vi "Action.vi"(8 "error in (no error)":errorcluster, 10 "OOQMH in":refnum<class "OOQMH.lvclass">, 11 "Get Notifiers in":refnum<class "Get Notifiers.lvclass">) -> (0 "error out":errorcluster, 2 "OOQMH out":refnum<class "OOQMH.lvclass">, 3 "Get Notifiers out":refnum<class "Get Notifiers.lvclass">)   [LabVIEW 2024, in "PID Loop.lvlib" / "Get Notifiers.lvclass"]
uses:
  Get Notifiers.lvclass
  Get Notifiers.lvclass/Get Notifiers.ctl
  PID Loop/PID Loop.lvclass
  C:/Users/uspoaotto/OneDrive - Oregon Tool/Desktop/working copies/helperLoop/src/OOQMH/OOQMH/OOQMH.lvclass
  C:/Users/uspoaotto/OneDrive - Oregon Tool/Desktop/working copies/helperLoop/src/PID Loop/PID Loop/PID Loop.lvclass
  OOQMH/OOQMH/OOQMH.lvclass
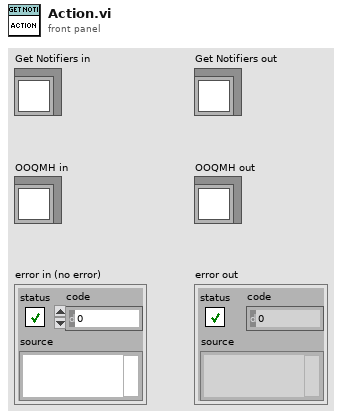
[diagram p1: front panel]
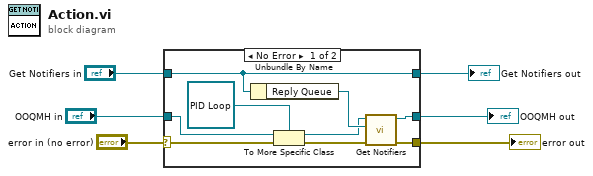
[diagram p0: block diagram]
diagram:
  n1 = case shown="No Error" "error in (no error)" {
    selector: "error in (no error)" -> [w8 w18]
    tunnel: [w9 w18] -> w5
    tunnel: [w11 w17] -> w4
    tunnel: "OOQMH in" -> [w14 w17]
    tunnel: "Get Notifiers in" -> [w7 w16]
    tunnel: [w7 w16] -> w1
    frame No Error {
      n2 = Unbundle By Name(w7) -> ("Reply Queue"=w15:refnum<queue>)
      n3 = To More Specific Class(target class=refnum<class "PID Loop.lvclass"> refnum ("PID Loop in"), reference=w14, error in=w8) -> (specific class reference=w12:refnum<class "PID Loop.lvclass">, error out=w10:errorcluster)
      n4 = call-dynamic "Get Notifiers.vi"("error in (no error)"=w10, "Reply Queue"=w15, "PID Loop in"=w12) -> ("error out"=w9:errorcluster, "PID Loop out"=w11:refnum<class "PID Loop.lvclass">)  [unwired: 7 in]
    }
    frame Error {
    }
  }
  "error out" <- w5
  "Get Notifiers out" <- w1
  "OOQMH out" <- w4
